vi "GetSomeData_GaGe4.vi"(0 "Handle Cluster":T1, 1 "tdms file":refnum<k34>, 2 "Save file?":bool, 3 "First chunk?":bool, 5 "Device":T2, 7 "Input settings":T5(array[cluster]), 11 "error in (no error)":errorcluster, 12 "Channel names in":string[](array[string])) -> (6 "Device out":T2, 8 "Input settings out":T5(array[cluster]), 10 "Data out":waveform(sgl)[](array[waveform]), 13 "Finished":bool, 14 "Channel names out":string[](array[string]), 15 "error out":errorcluster)   [LabVIEW 2015]
doc: "DESCRIPTION:\nThis VI retrieves the specified amount of data from one or more analog input channels each time a digital start trigger, digital stop trigger, or digital start and stop trigger, occur. It shows how to trigger an acquisition multiple times while avoiding the overhead of configuration and buffer allocation each time. This is a timed acquisition, meaning that a hardware clock is used to control the acquisition rate for fast and accurate timing. It is also a buffered acquisition, meaning that the data are stored in an intermediate memory buffer after they are acquired from the DAQ board. When the pretrigger scans is set to 0, you must set \"choose trigger type\" to START OR STOP TRIGGER (and use a start trigger). Your start trigger will then start your DAQ board and acquisition into a buffer to be read by LabVIEW. When the pretrigger scans is set to greater than 1, you can set \"choose trigger type\" to START OR STOP TRIGGER (and use a stop trigger) or START & STOP TRIGGER (and use both). If you use only the stop trigger, a software strobe starts your DAQ board and your stop trigger will determine when data are acquired into a buffer to be read by LabVIEW. If you use a start and stop trigger, your start trigger will start the DAQ board, but your stop trigger will determine when data are acquired into a buffer to be read by LabVIEW. In either case, your pretrigger scans will be the number of scans to acquire before the stop trigger occurs. The rest of the number of scans to acquire will be after the stop trigger. Data are retrieved from that buffer and displayed after the appropriate amount (before and after the stop trigger) have been acquired. The vertical cursor on the graph indicates where the trigger occurred. With each iteration of the while loop, the VI waits for the next trigger, then reads the same amount of data again from the same channels at the same rate.\n\nUse this VI to wait for multiple digital triggers, acquiring a relatively small amount of data for each trigger (it must fit in the memory available), where each point does not need to be viewed or processed while it is being acquired\n\nINSTRUCTIONS:\n1. Enter the device number, channels, number of scans to acquire, and scan rate.\n2. Enter the pretrigger scans, trigger edge, and time limit.\n3. Set choose trigger type to START OR STOP TRIGGER (to hardware start) if pretrigger scans = 0, If pretrigger scans > 0, set it to START OR STOP TRIGGER (to software start and hardware stop) or START & STOP TRIGGER (to hardware start and hardware stop).\n4. Make the appropriate I/O connections as explained below.\n5. Run the VI.\n\nKEY PARAMETERS:\nThis VI shows how to use the intermediate analog input DAQ VIs to trigger multiple acquisitions. \n\nAI Config.vi is only called on the first iteration of the while loop. This avoids the overhead of configuration and buffer allocation for each acquisition. However, you must stop and restart the VI if you wish to change input parameters.\n\nThe \"read/search mode\" for AI Read.vi is set to \"relative to trigger point\", since this is a hardware triggered acquisition. \n\nAI Control.vi (an advanced analog input VI) is called, in the event that AI Read.vi times out, to momentarily stop the analog input clock. This is needed so the input clock is not running when AI Start.vi (which restarts the clock) is called again.\n\nI/O CONNECTIONS:\nConnect to the input channels on the I/O connector for your board to match the channels you have chosen on the front panel of this VI. For example ACH0 for analog input.\n\nE series boards:\nConnect your start trigger to PFI0/TRIG1, your stop trigger to PFI1/TRIG2.\n\nLegacy MIO boards:\nConnect your start trigger to STARTRIG*, your stop trigger to STOPTRIG.\n\nLegacy MIO-16X, MIO-16F-5, and MIO-64F-5:\nThe start and stop trigger pin is EXTTRIG*.\n\nLab/1200 series boards:\nConnect your start or stop trigger to EXTTRIG. Hardware pretriggering (start & stop) is not supported.\n\nThe PC-LPM-16, DAQCard-500, and DAQCard-700 are not supported by this example.\n\nTo find the actual pin numbers, refer to your hardware user manual.\n\nDAQ VIs USED:\nAI Config.vi, AI Start.vi, AI Read.vi, AI Control.vi, AI Clear.vi."
uses:
  CompuScope_LabVIEW_SDK/CsLv/CsLV.dll
panel:
  out "Depth":dbl
  out "Segment Size":dbl
  out "Timing out":T3
  in  "Trigger and sampling":T4={"Trig. edge"=enum."Falling", "Trig. source"=enum."External", "Trig. level"=2.0, "Oversample"=FALSE, "Oversamplie by"=1, "Average samples"=TRUE, "Oversample\nto match rates"=FALSE} {"Trig. level" format="%.2f"}
  in  "Timing":T3
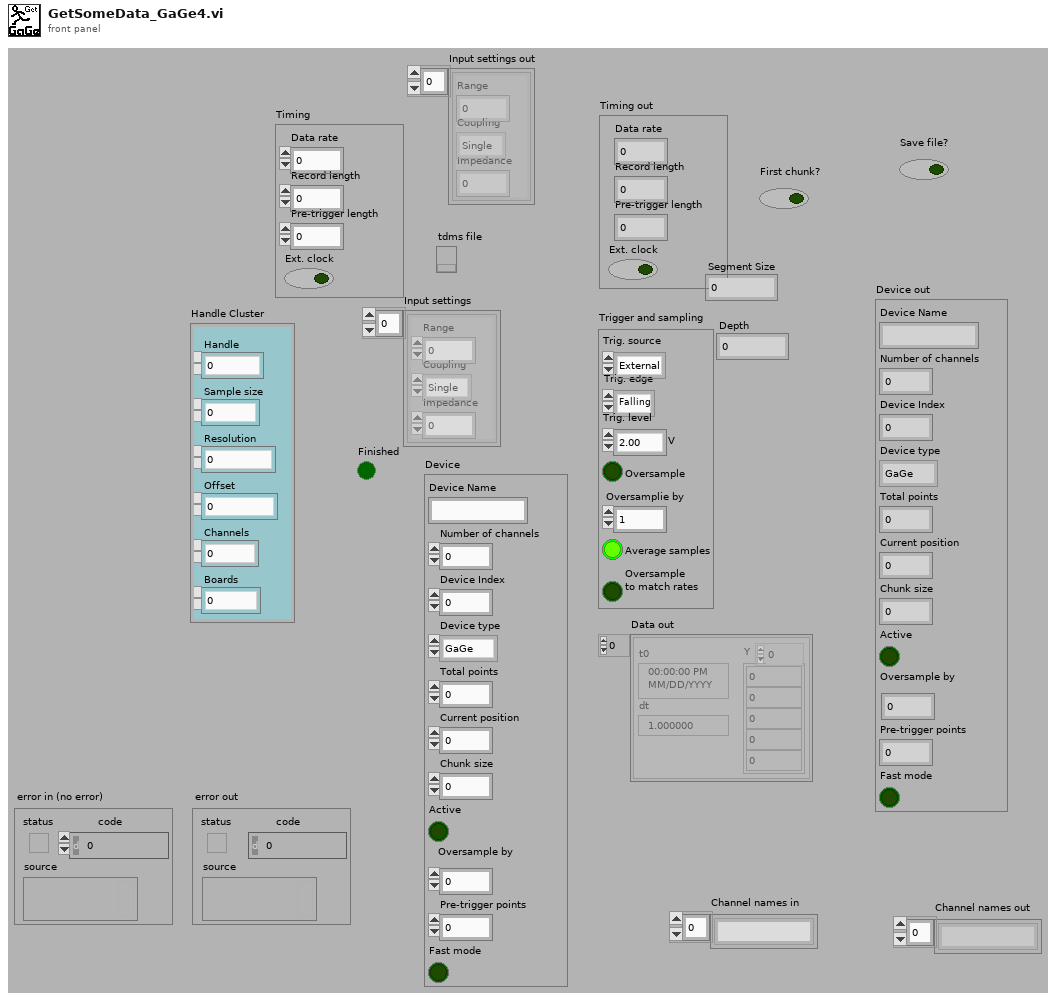
[diagram p1: front panel]
types:
  T1 = cluster{"Handle":u32, "Sample size":u32, "Resolution":i32, "Offset":i32, "Channels":u32, "Boards":u32}
  T2 = cluster{"Device Name":string, "Number of channels":i32, "Device Index":i32, "Device type":enum16{"GaGe", "NI-DAQ", "NI-Scope", "CAMAC", "VXI-1433", "VXI-1437"}, "Total points":i64, "Current position":i64, "Chunk size":i64, "Active":bool, "Oversample by":i32, "Pre-trigger points":i64, "Fast mode":bool}
  T3 = cluster{"Data rate":dbl, "Record length":dbl, "Pre-trigger length":dbl, "Ext. clock":bool}
  T4 = cluster{"Trig. edge":enum16{"Rising", "Falling"}, "Trig. source":enum16{"External", "Immediate"}, "Trig. level":sgl[unit], "Oversample":bool, "Oversamplie by":i32, "Average samples":bool, "Oversample\nto match rates":bool}
  T5 = cluster{"Range":dbl, "Coupling":enum16{"Single", "Differen"}, "Impedance":dbl}[]
  T6 = cluster{"Handle":u32, "Sample Size":u32, "Resolution":i32, "Offset":i32, "Channels":u32, "Boards":u32}
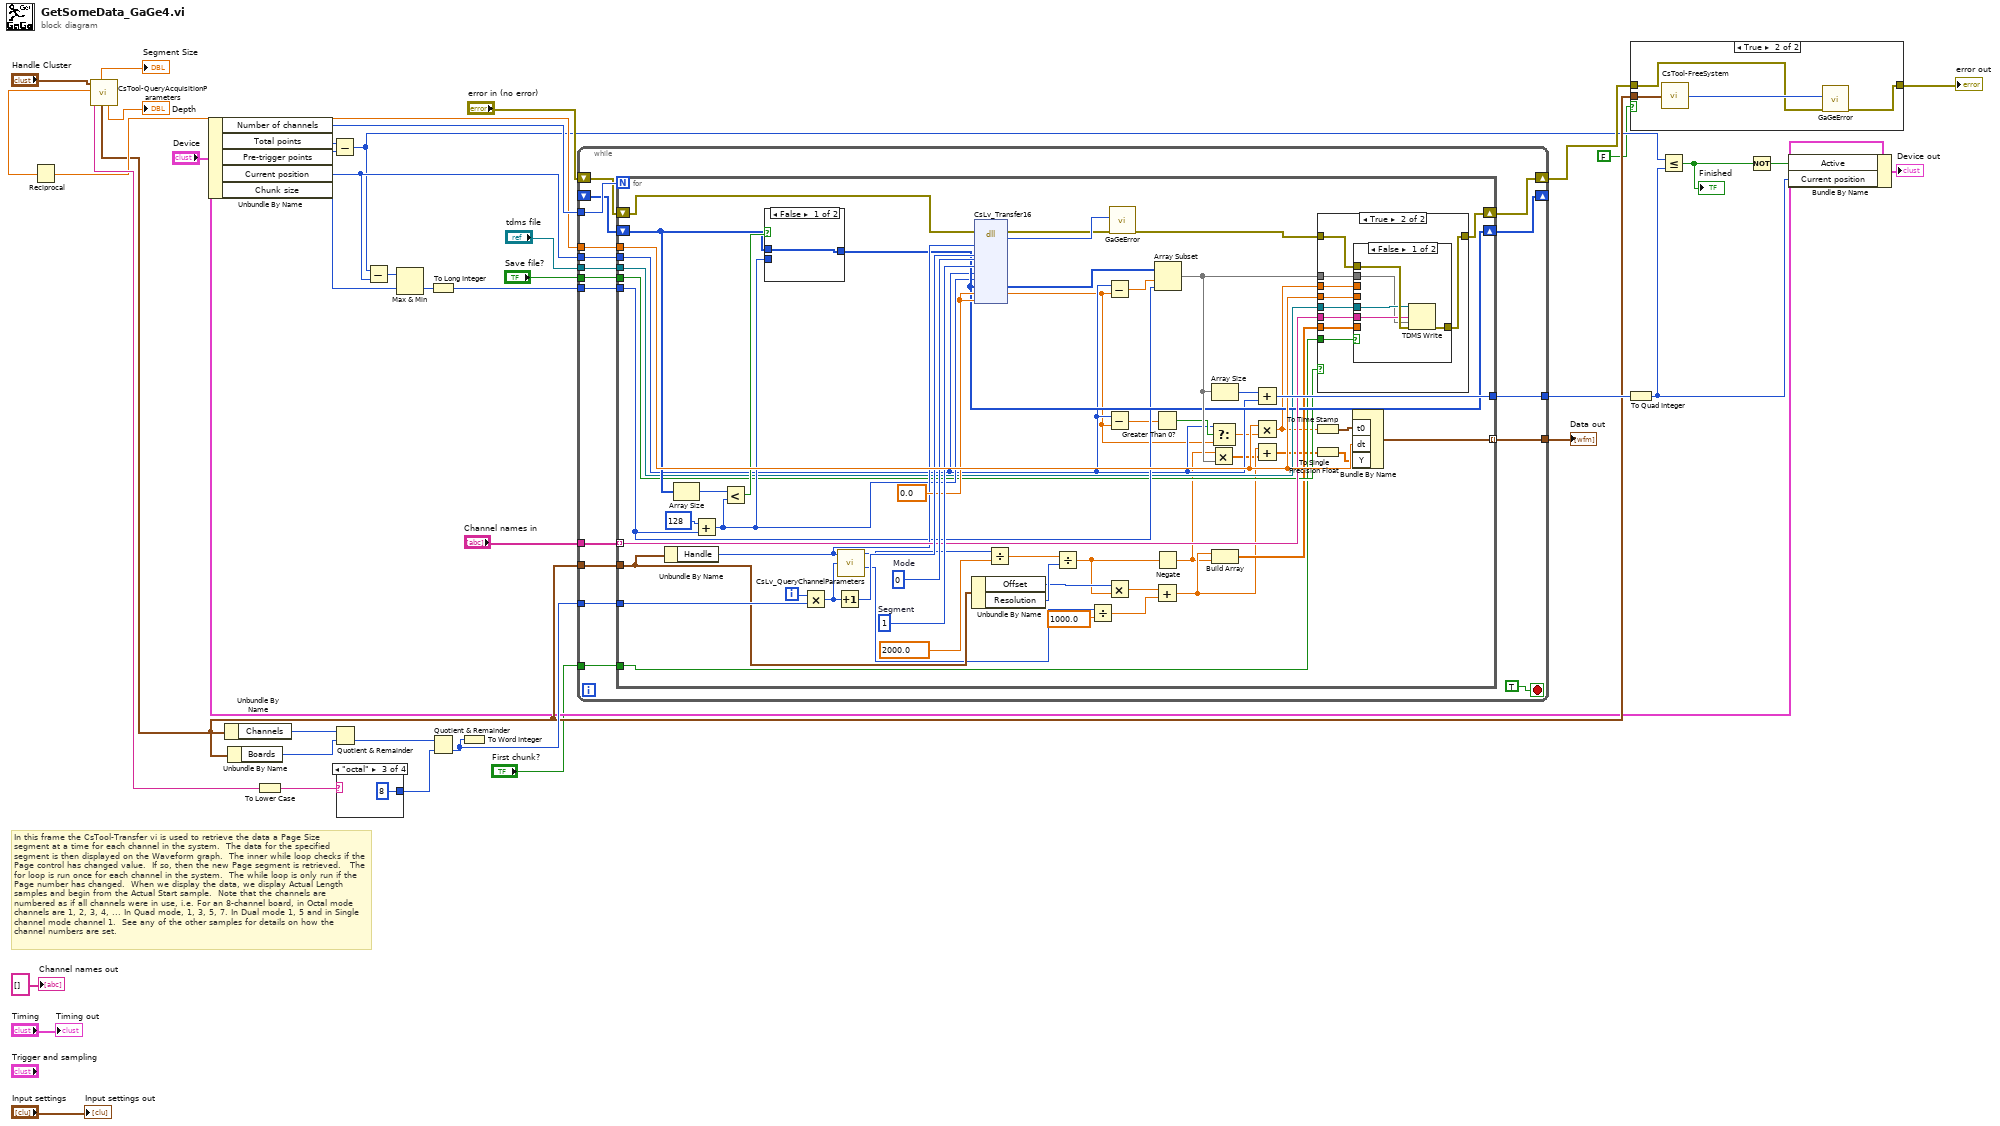
[diagram p0: block diagram]
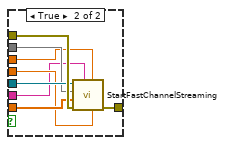
[diagram p3: hidden frame]
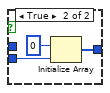
[diagram p4: hidden frame]
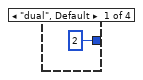
[diagram p5: hidden frame]
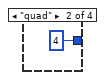
[diagram p6: hidden frame]
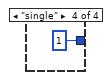
[diagram p7: hidden frame]
diagram:
  # "In this frame the CsTool-Transfer vi is used to retrieve the data a Page Size \nsegment at a time for each channel in the system.  The data for the specified segment is then displayed on the Waveform graph.  The inner while loop checks if the Page control has changed value.  If so, then the new Page segment is retrieved.   The for loop is run once for each channel in the system.  The while loop is only run if the Page number has changed.  When we display the data, we display Actual Length samples and begin from the Actual Start sample.  Note that the channels are numbered as if all channels were in use, i.e. For an 8-channel board, in Octal mode channels are 1, 2, 3, 4, ... In Quad mode, 1, 3, 5, 7. In Dual mode 1, 5 and in Single channel mode channel 1.  See any of the other samples for details on how the channel numbers are set."
  n1 = call "CsTool-QueryAcquisitionParameters.vi"("Handle Cluster"="Handle Cluster") -> ("Depth"=→"Depth":dbl, "Output Handle Cluster"=w15:T6, "Segment Size"=→"Segment Size":dbl, "Mode"=w32:string, "Sample Rate"=w22:dbl)  [unwired: 6 out]
  n2 = Reciprocal(x=w22) -> (1/x=w23:dbl)
  n3 = Unbundle By Name("Device") -> ("Number of channels"=w24:i32, "Total points"=w36:i64, "Pre-trigger points"=w13:i64, "Current position"=w21:i64, "Chunk size"=w25:i64)
  n4 = Unbundle By Name(w15) -> ("Channels"=w27:u32)
  n5 = Unbundle By Name(w15) -> ("Boards"=w30:u32)
  n6 = To Lower Case(string=w32) -> (all lower case string=w31:string)
  n7 = Subtract(x=w36, y=w13) -> (x-y=w14:i64)
  n8 = Quotient & Remainder(x=w27, y=w30) -> (floor(x/y)=w29:u32)  [unwired: 1 out]
  n9 = case shown="\"octal\"" w31 {
    tunnel: [2 4 8 1] -> w28
    frame "dual", Default {
    }
    frame "quad" {
    }
    frame "octal" {
    }
    frame "single" {
    }
  }
  n10 = Subtract(x=w14, y=w21) -> (x-y=w38:i64)
  n11 = Max & Min(x=w38, y=w25) -> (min(x,y)=w39:i64)  [unwired: 1 out]
  n12 = To Long Integer(number=w39) -> (32bit integer=w20:i32)
  n13 = Quotient & Remainder(x=w29, y=w28) -> (floor(x/y)=w26:u32)  [unwired: 1 out]
  n14 = To Word Integer(number=w26) -> ()  [unwired: 1 out]
  n15 = while {
    tunnel: w26 -> [w61]
    tunnel: w24 -> [w60]
    tunnel: w23 -> [w59]
    tunnel: w21 -> [w58]
    tunnel: w20 -> [w57]
    tunnel: [w56] -> w18
    tunnel: w15 -> [w53]
    tunnel: "Channel names in" -> [w52]
    shift-right: [w54] -> w16
    shift-left: "error in (no error)" -> [w55]
    shift-right: [w51] -> _
    shift-left: _ -> [w50]
    tunnel: "tdms file" -> [w48]
    tunnel: "Save file?" -> [w47]
    tunnel: "First chunk?" -> [w46]
    tunnel: [w45] -> w19
    stop <- TRUE stop-if-true
    n16 = for {
      N: w60 -> [_]
      tunnel: w53 -> [w99]
      tunnel: w61 -> [w115]
      tunnel: w59 -> [w113]
      tunnel: w58 -> [w82]
      tunnel: w57 -> [w91]
      tunnel: [w114] -> w56
      shift-right: [w103] -> w54
      shift-left: w55 -> [w90]
      tunnel: w52 -> [w102] mode=indexing
      shift-right: [w96] -> w51
      shift-left: w50 -> [w92]
      tunnel: w47 -> [w87]
      tunnel: w46 -> [w86]
      tunnel: [w85] -> w45 mode=indexing
      tunnel: w48 -> [w88]
      i -> [w116]
      w108 = 0.0
      w109 = u32 1  # Segment
      w110 = u32 0  # Mode
      n17 = Unbundle By Name(w99) -> ("Handle"=w101:u32)
      n18 = Array Size(array=w92) -> (size(s)=w93:i32)
      n19 = Add(x=128, y=w91) -> (x+y=w94:i32)
      n20 = Less?(x=w93, y=w94) -> (x < y?=w95:bool)
      n21 = case shown="False" w95 {
        tunnel: w94 -> [_ w143]
        tunnel: [w140 w141] -> w96
        tunnel: w92 -> [w140 _]
        frame False {
        }
        frame True {
          n22 = Initialize Array(i16 0 ("element"), w143) -> (w141:i16[])
        }
      }
      n23 = Multiply(x=w116, y=w115) -> (x*y=w100:u32)
      n24 = Increment(x=w100) -> (x+1=w111:u32)
      n25 = call "CsLv_QueryChannelParameters.vi"("Channel"=w100, "Handle"=w101) -> ("DC Offset (mV)"=w77:i32, "Input Range (mV)"=w76:u32)  [unwired: 5 out]
      n26 = Unbundle By Name(w99) -> ("Offset"=w73:i32, "Resolution"=w75:i32)
      n27 = dll-call lib="D:/github/DAQ/Libraries/GaGe-DAQ/CompuScope_LabVIEW_SDK/CsLv/CsLV.dll" fn="CsLv_Transfer16"(error in=w90, "Handle"=w101, "Channel"=w111, "Segment"=w110, "Mode"=w109, "Start"=w82, "Length"=w94, "Buffer"=w96, "ActualStart"=w108, "ActualLength"=w108) -> (error out=w89:errorcluster, w107:i32, "Buffer"=w105:i16[], "ActualStart"=w81:dbl)  [unwired: 5 in, 5 out]
      n28 = Divide(x=w76, y=2000.0) -> (x/y=w74:dbl)
      n29 = Divide(x=w74, y=w75) -> (x/y=w70:dbl)
      n30 = Divide(x=w77, y=1000.0) -> (x/y=w71:dbl)
      n31 = Subtract(x=w82, y=w81) -> (x-y=w106:dbl)
      n32 = Subtract(x=w82, y=w81) -> (x-y=w84:dbl)
      n33 = Multiply(x=w73, y=w70) -> (x*y=w72:dbl)
      n34 = call "GaGeError.vi"("error in (no error)"=w89, "Error Code"=w107) -> ("error out"=w104:errorcluster)  [unwired: 4 in, 5 out]
      n35 = Greater Than 0?(x=w84) -> (x > 0?=w83:bool)
      n36 = Add(x=w72, y=w71) -> (x+y=w65:dbl)
      n37 = Array Subset(array=w105, index=w106, length=w91) -> (w98:i16[])
      n38 = Negate(x=w70) -> (-x=w64:dbl)
      n39 = Multiply(x=w64, y=w98) -> (x*y=w63:dbl[])
      n40 = Select(t=w82, s=w83, f=w81) -> (s? t:f=w80:dbl)
      n41 = Array Size(array=w98) -> (size(s)=w97:i32)
      n42 = Build Array(w65, w64) -> (w69:dbl[])
      n43 = Add(x=w97, y=w82) -> (x+y=w114:i64)
      n44 = Multiply(x=w113, y=w80) -> (x*y=w62:dbl)
      n45 = Add(x=w65, y=w63) -> (x+y=w67:dbl[])
      n46 = To Time Stamp(1:w62) -> (0:w66:timestamp)
      n47 = To Single Precision Float(number=w67) -> (single precision float=w68:sgl[])
      n48 = case shown="True" w87 {
        tunnel: [w117 w126] -> w103
        tunnel: w104 -> [w117 w125]
        tunnel: w88 -> [_ w124]
        tunnel: w98 -> [_ w123]
        tunnel: w69 -> [_ w122]
        tunnel: w113 -> [_ w121]
        tunnel: w102 -> [_ w120]
        tunnel: w62 -> [_ w119]
        tunnel: w86 -> [_ w118]
        frame False {
        }
        frame True {
          n49 = case shown="False" w118 {
            tunnel: [w130 w139] -> w126
            tunnel: w125 -> [w131 w138]
            tunnel: w124 -> [w129 w137]
            tunnel: w123 -> [w127 w136]
            tunnel: w122 -> [_ w135]
            tunnel: w121 -> [_ w134]
            tunnel: w120 -> [w128 w133]
            tunnel: w119 -> [_ w132]
            frame False {
              n50 = TDMS Write(0:w129, 7:w128, 9:w127, 11:w131) -> (15:w130:errorcluster)  [unwired: 2 in, 3 out]
            }
            frame True {
              n51 = call "StartFastChannelStreaming.vi"("dt"=w134, "t0"=w132, "channel name(s) in (Untitled)"=w133, "error in (no error)"=w138, "Scaling coefficients"=w135, "Data"=w136, "tdms file"=w137) -> ("error out"=w139:errorcluster)  [unwired: 1 in, 3 out]
            }
          }
        }
      }
      n52 = Bundle By Name("t0"=w66, "dt"=w113, "Y"=w68) -> (w85:waveform(sgl))  [unwired: 1 out]
    }
  }
  "Data out" <- w19
  n53 = To Quad Integer(1:w18) -> (0:w33:i64)
  n54 = case shown="True" FALSE {
    tunnel: [w144 w145] -> w40
    tunnel: w16 -> [w144 w146]
    tunnel: w15 -> [_ w148]
    frame False {
    }
    frame True {
      n55 = call "CsTool-FreeSystem.vi"("Handle Cluster"=w148) -> ("Error Code"=w147:i32)
      n56 = call "GaGeError.vi"("error in (no error)"=w146, "Error Code"=w147) -> ("error out"=w145:errorcluster)  [unwired: 4 in, 5 out]
    }
  }
  "error out" <- w40
  n57 = Less Or Equal?(x=w14, y=w33) -> (x <= y?=w11:bool)
  "Finished" <- w11
  n58 = Not(x=w11) -> (.not. x?=w12:bool)
  n59 = Bundle By Name(cluster="Device", "Active"=w12, "Current position"=w33) -> (→"Device out":T2)
  "Input settings out" <- "Input settings"
  "Timing out" <- "Timing"
  "Channel names out" <- string[] [] ("Channel names in")
